vi "FTW-Router-Destroy.vi"(0 "FTW Router":refnum<class "FTW-Router.lvclass">, 11 "error in":errorcluster) -> (15 "error out":errorcluster)   [LabVIEW 2013, in "FTW-Actor.lvlib" / "FTW-Router.lvclass"]
uses:
  FTW-Router.lvclass
  Endpoint/FTW-Endpoint.lvclass
panel:
  # "Inputs"
  # "Outputs"
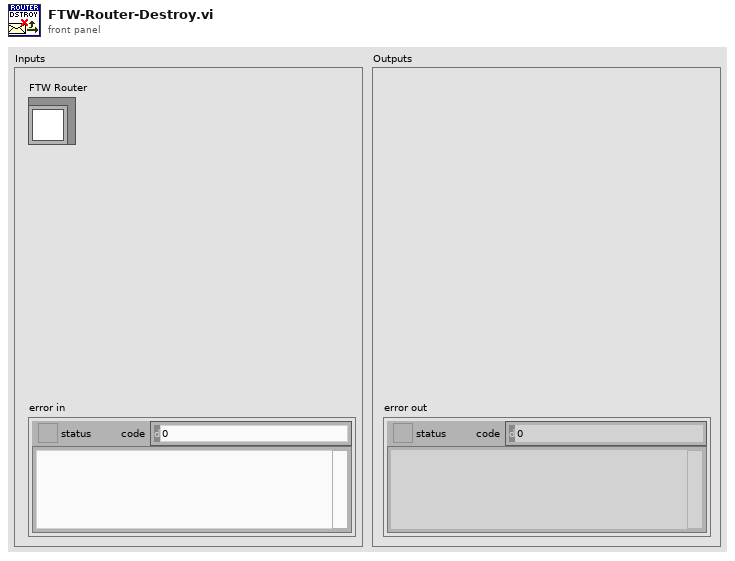
[diagram p1: front panel]
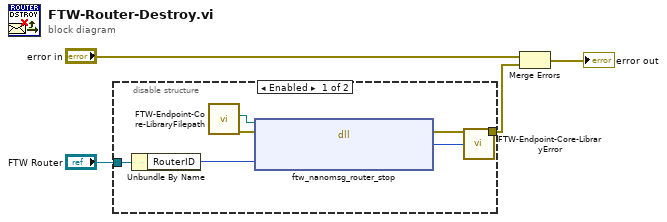
[diagram p0: block diagram]
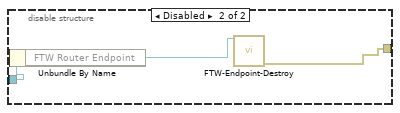
[diagram p2: hidden frame]
diagram:
  n1 = disable-structure shown="Enabled" {
    disable-tunnel: [w7 w12] -> w3
    disable-tunnel: "FTW Router" -> [w6 w14]
    frame Enabled {
      n2 = Unbundle By Name(w6) -> ("RouterID"=w5:i64)
      n3 = call "FTW-Endpoint-Core-LibraryFilepath.vi"() -> ("error out"=w8:errorcluster, "Library Filepath"=w11:path)  [unwired: 9 in, 1 out]
      n4 = dll-call lib="C:/Users/Jack/repo/ftw-master/Actor/src/Endpoint/Core/FTWLib-nanomsg32.dll" fn="ftw_nanomsg_router_stop"(path in=w11, error in=w8, "RouterID"=w5) -> (error out=w10:errorcluster, "Return Value"=w9:i64)  [unwired: 2 in, 1 out]
      n5 = call "FTW-Endpoint-Core-LibraryError.vi"("error in"=w10, "Return Value"=w9) -> ("error out"=w7:errorcluster)  [unwired: 13 in]
    }
    frame Disabled {
      n6 = Unbundle By Name(w14) -> ("FTW Router Endpoint"=w13:refnum<class "FTW-Endpoint.lvclass">)
      n7 = call-dynamic "FTW-Endpoint-Destroy.vi"("FTW Socket"=w13) -> ("error out"=w12:errorcluster)  [unwired: 14 in]
    }
  }
  n8 = Merge Errors("error in", w3) -> (→"error out":errorcluster)
